vi "Main.vi"() -> ()   [LabVIEW 2018]
panel:
  out "Good Packet":bool
  out "Return Value":string
  in  "ADC":bool
  out "error out":errorcluster
  out "remote port":u16
  out "remote address":string
  in  "1":bool
  in  "0":bool
  in  "PRIGAIN":dbl format="%.3f"
  in  "CODERATE":u8
  out "bytes written":i32
  out "x > y?":bool
  out "SENT":string
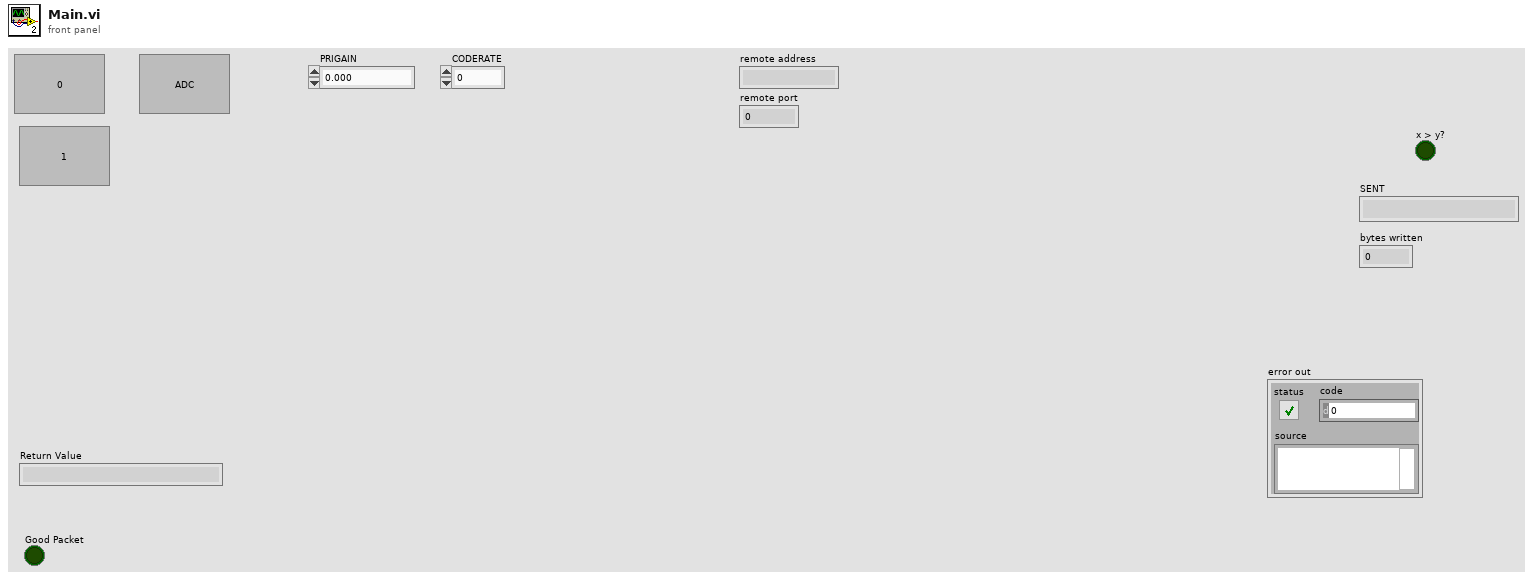
[diagram p1: front panel]
types:
  T1 = enum16{"Standard", "Buffered", "CRLF", "Immediate"}
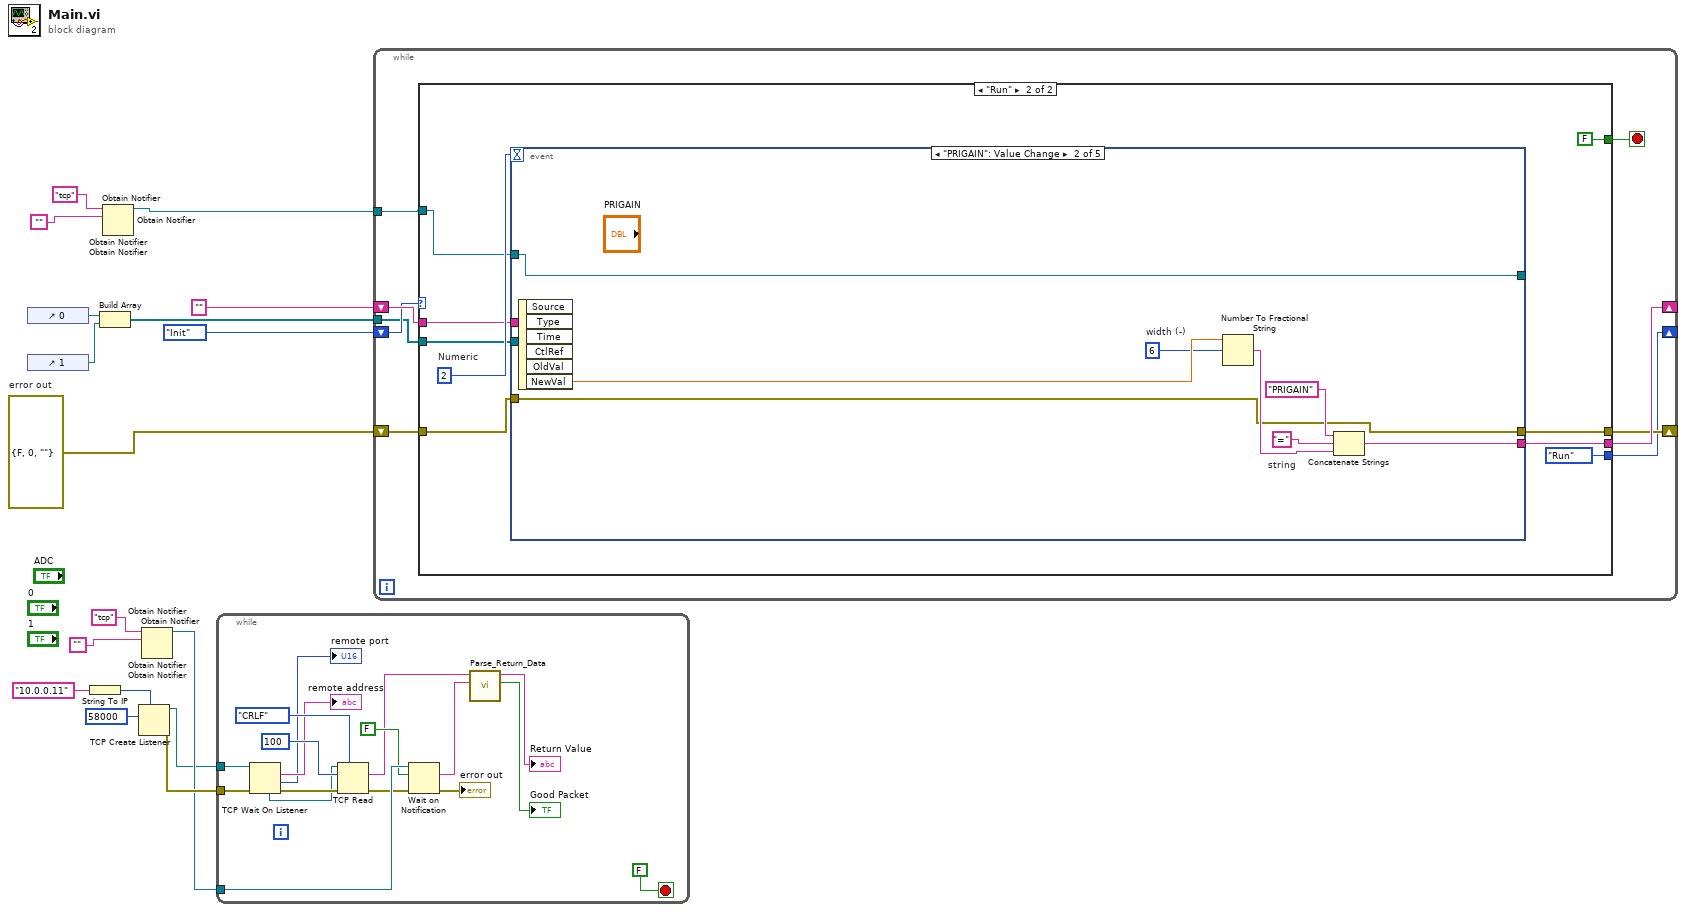
[diagram p0: block diagram]
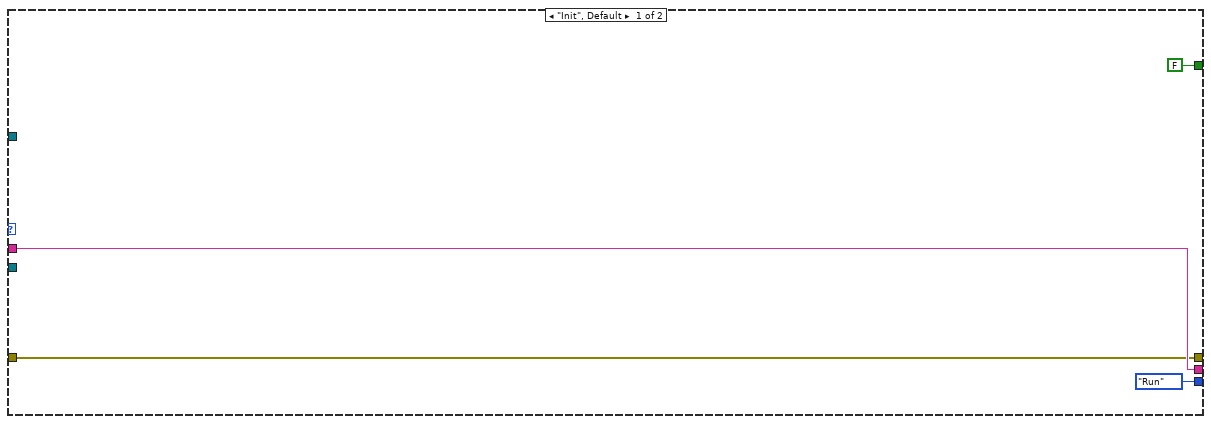
[diagram p2: hidden frame]
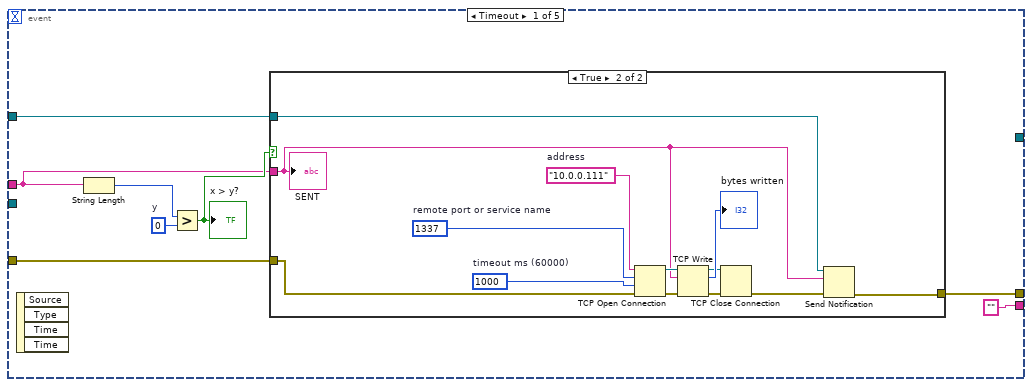
[diagram p3: hidden frame]
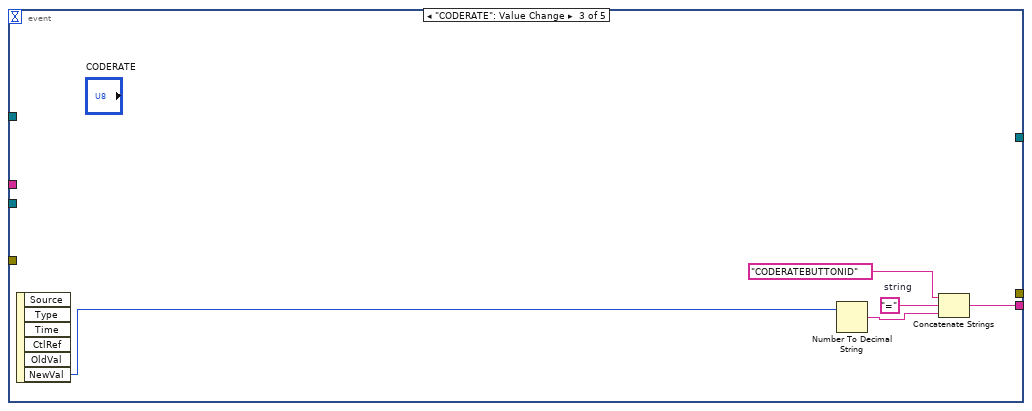
[diagram p5: hidden frame]
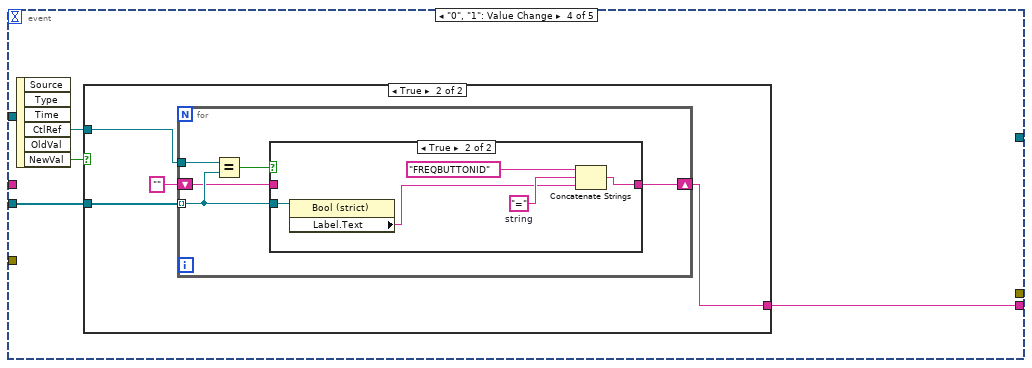
[diagram p6: hidden frame]
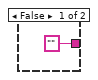
[diagram p7: hidden frame]
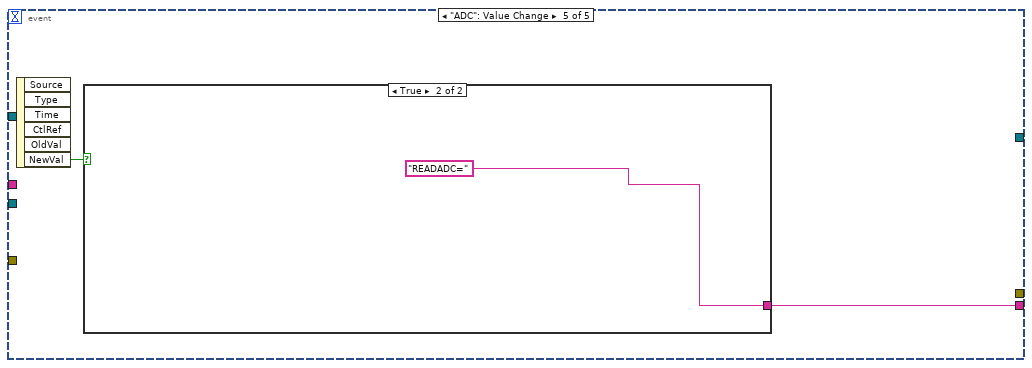
[diagram p9: hidden frame]
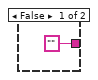
[diagram p10: hidden frame]
diagram:
  w28 = errorcluster {"status"=FALSE, "code"=0, "source"=""}  # error out
  n1 = control-ref of="0"() -> (w25:refnum<vi>)
  n2 = control-ref of="1"() -> (w24:refnum<vi>)
  n3 = String To IP(1:"10.0.0.11" ("name")) -> (0:w21:u32)
  n4 = Build Array(w25, w24) -> (w26:refnum<vi>[])
  n5 = Obtain Notifier(name (unnamed)="tcp", notification data type="") -> ()  [unwired: 2 in, 3 out]
  n6 = Obtain Notifier(name (unnamed)="tcp", notification data type="") -> ()  [unwired: 2 in, 3 out]
  n7 = Obtain Notifier(name (unnamed)="tcp", notification data type="") -> ()  [unwired: 2 in, 3 out]
  n8 = Obtain Notifier(name (unnamed)="tcp", notification data type="") -> (notifier out=w2:refnum<notifier>)  [unwired: 2 in, 2 out]
  n9 = TCP Create Listener(7:w21, 10:u16 58000 ("port")) -> (0:w20:errorcluster, 3:w1:refnum<k5>)  [unwired: 3 in, 1 out]
  n10 = Obtain Notifier(name (unnamed)="tcp", notification data type="") -> (notifier out=w3:refnum<notifier>)  [unwired: 2 in, 2 out]
  n11 = Obtain Notifier(name (unnamed)="tcp", notification data type="") -> ()  [unwired: 2 in, 3 out]
  n12 = Obtain Notifier(name (unnamed)="tcp", notification data type="") -> ()  [unwired: 2 in, 3 out]
  n13 = Obtain Notifier(name (unnamed)="tcp", notification data type="") -> ()  [unwired: 2 in, 3 out]
  n14 = while {
    tunnel: w20 -> [w39]
    tunnel: w3 -> [w37]
    tunnel: w1 -> [w38]
    stop <- FALSE stop-if-true
    n15 = TCP Wait On Listener(8:w39, 11:w38) -> (0:w43:errorcluster, 1:→"remote port":u16, 2:→"remote address":string, 4:w40:refnum<k5>)  [unwired: 2 in, 1 out]
    n16 = TCP Read(connection ID=w40, bytes to read=100, error in (no error)=w43, 7:T1."CRLF" ("mode (standard)")) -> (data out=w32:string, error out=w35:errorcluster)  [unwired: 1 in, 1 out]
    n17 = Wait on Notification(notifier=w37, ignore previous (F)=FALSE, error in (no error)=w35) -> (notification=w33:string, error out=→"error out":errorcluster)  [unwired: 1 in, 2 out]
    n18 = call "Parse_Return_Data.vi"("String"=w33, "data in"=w32) -> ("x = y?"=→"Good Packet":bool, "Return Value"=→"Return Value":string)  [unwired: 6 in, 2 out]
  }
  n19 = while {
    shift-right: [w55] -> _
    shift-left: "" -> [w54]
    shift-right: [w53] -> _
    shift-left: w28 -> [w52]
    shift-right: [w50] -> _
    shift-left: enum16{"Init", "Run"}."Init" -> [w49]
    tunnel: w26 -> [w48]
    tunnel: w2 -> [w47]
    stop <- w51 stop-if-true
    n20 = case shown="\"Run\"" w49 {
      tunnel: [FALSE FALSE] -> w51
      tunnel: [w57 w66] -> w55
      tunnel: w54 -> [w57 w65]
      tunnel: [w56 w64] -> w53
      tunnel: w52 -> [w56 w63]
      tunnel: [enum16{"Init", "Run"}."Run" enum16{"Init", "Run"}."Run"] -> w50
      tunnel: w48 -> [_ w61]
      tunnel: w47 -> [_ w60]
      frame "Init", Default {
      }
      frame "Run" {
        w68 = 2  # Numeric
        n21 = event shown="[1] \"PRIGAIN\": Value Change" {
          selector: _ -> [_ _ _ _ _]
          dyn-events: _ -> [_ _ _ _ _]
          timeout: w68 -> [_ _ _ _ _]
          tunnel: ["" w96 w101 w105 w125] -> w66
          tunnel: w65 -> [w73 _ _ _ _]
          tunnel: [w71 w91 _ _ _] -> w64
          tunnel: w63 -> [w70 w91 _ _ _]
          tunnel: w61 -> [_ _ _ w107 _]
          tunnel: [_ w92 _ _ _] -> _
          tunnel: w60 -> [w69 w92 _ _ _]
          event Timeout {
            w75 = 0  # y
            n22 = event-data() -> ()  [unwired: 1 in, 4 out]
            n23 = String Length(string=w73) -> (length=w76:i32)
            n24 = Greater?(x=w76, y=w75) -> (0:w74:bool)
            "x > y?" <- w74
            n25 = case shown="True" w74 {
              tunnel: w73 -> [_ w78]
              tunnel: [w77 w80] -> w71
              tunnel: w70 -> [w77 w87]
              tunnel: w69 -> [_ w79]
              frame False {
              }
              frame True {
                w85 = 1000  # timeout ms (60000)
                w86 = u16 1337  # remote port or service name
                w90 = "10.0.0.111"  # address
                n26 = TCP Open Connection(address=w90, remote port or service name=w86, timeout ms (60000)=w85, error in (no error)=w87) -> (connection ID=w89:refnum<k5>, error out=w88:errorcluster)  [unwired: 1 in]
                n27 = TCP Write(connection ID=w89, data in=w78, error in (no error)=w88) -> (connection ID out=w82:refnum<k5>, bytes written=→"bytes written":i32, error out=w83:errorcluster)  [unwired: 1 in]
                n28 = TCP Close Connection(connection ID=w82, error in (no error)=w83) -> (error out=w81:errorcluster)  [unwired: 1 in, 1 out]
                n29 = Send Notification(notification=w78, notifier=w79, error in (no error)=w81) -> (error out=w80:errorcluster)  [unwired: 1 out]
                "SENT" <- w78
              }
            }
          }
          event "PRIGAIN": Value Change {
            w93 = i16 6  # width (-)
            w94 = "="  # string
            n30 = event-data() -> ("NewVal"=w98:dbl)  [unwired: 1 in, 5 out]
            n31 = Number To Fractional String(number=w98, width (-)=w93) -> (F-format string=w95:string)  [unwired: 2 in]
            n32 = Concatenate Strings("PRIGAIN", w94, w95) -> (w96:string)
          }
          event "CODERATE": Value Change {
            w100 = "="  # string
            n33 = event-data() -> ("NewVal"=w102:u8)  [unwired: 1 in, 5 out]
            n34 = Number To Decimal String(number=w102) -> (decimal integer string=w99:string)  [unwired: 1 in]
            n35 = Concatenate Strings("CODERATEBUTTONID", w100, w99) -> (w101:string)
          }
          event "0", "1": Value Change {
            n36 = event-data() -> ("CtlRef"=w106:refnum<vi>, "NewVal"=w104:bool)  [unwired: 1 in, 4 out]
            n37 = case shown="True" w104 {
              tunnel: w107 -> [_ w112]
              tunnel: w106 -> [_ w111]
              tunnel: ["" w110] -> w105
              frame False {
              }
              frame True {
                n38 = for {
                  tunnel: w111 -> [w117]
                  tunnel: w112 -> [w115] mode=indexing
                  shift-right: [w114] -> w110
                  shift-left: "" -> [w113]
                  n39 = Equal?(x=w117, y=w115) -> (x = y?=w116:bool)
                  n40 = case shown="True" w116 {
                    tunnel: w115 -> [_ w123]
                    tunnel: [w118 w120] -> w114
                    tunnel: w113 -> [w118 _]
                    frame False {
                    }
                    frame True {
                      w121 = "="  # string
                      n41 = property class="Bool (strict)"(reference=w123) -> ("Label.Text"=w119:string)  [unwired: 1 in, 2 out]
                      n42 = Concatenate Strings("FREQBUTTONID", w121, w119) -> (w120:string)
                    }
                  }
                }
              }
            }
          }
          event "ADC": Value Change {
            n43 = event-data() -> ("NewVal"=w124:bool)  [unwired: 1 in, 5 out]
            n44 = case shown="True" w124 {
              tunnel: ["" "READADC="] -> w125
              frame False {
              }
              frame True {
              }
            }
          }
        }
      }
    }
  }
